vi "Menu.vi"() -> ()   [LabVIEW 2025]
panel:
  in  "Tab Control":enum32{"Page 1", "Page 2"}(tab)
  in  "Start Game":bool
  in  "Exit":bool
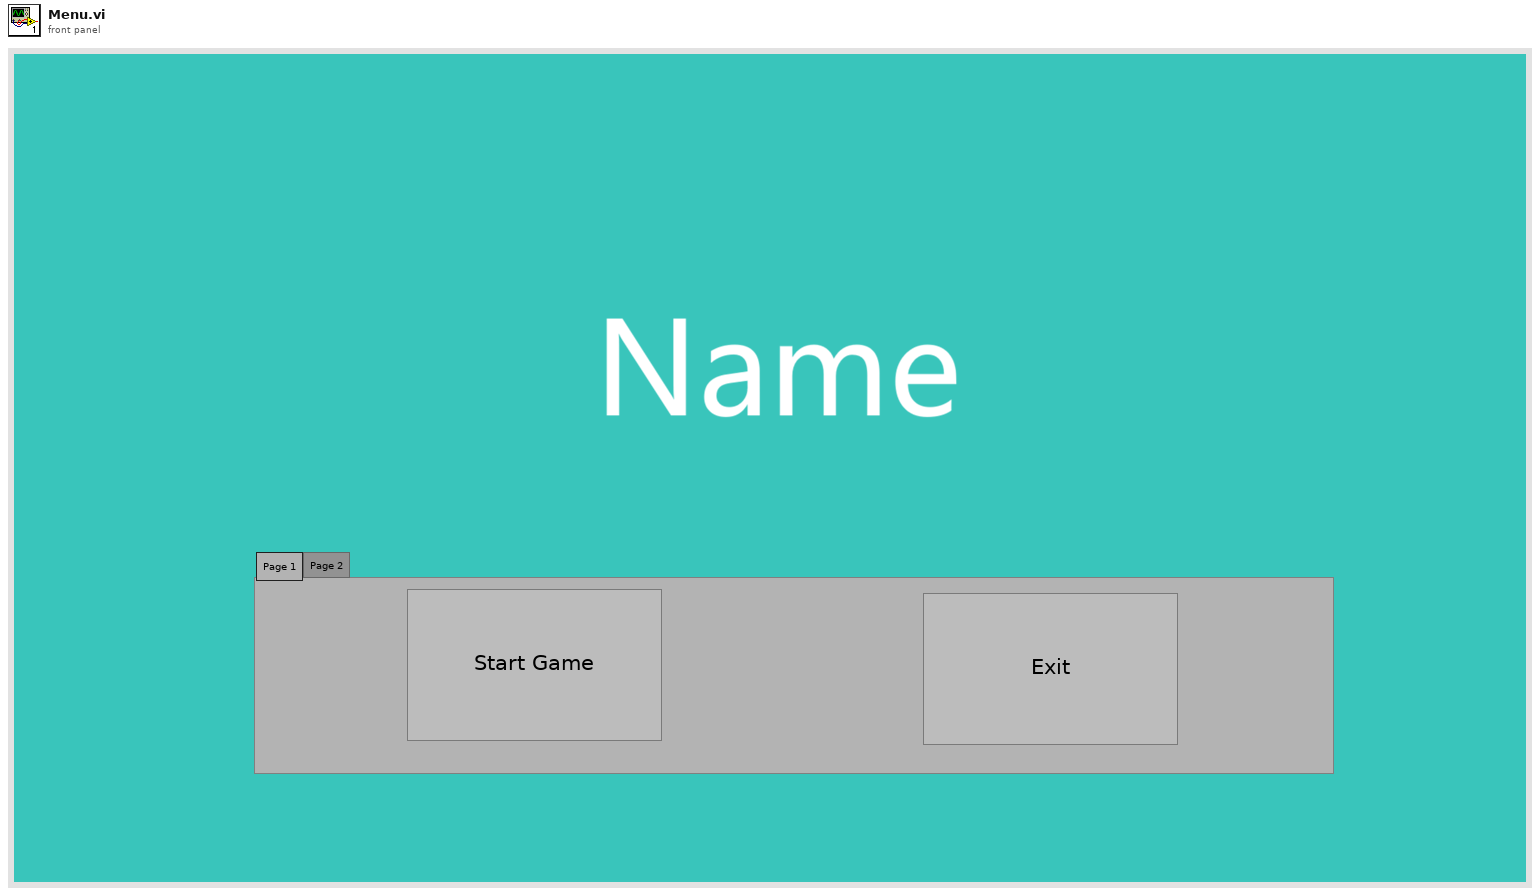
[diagram p1: front panel]
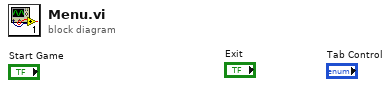
[diagram p0: block diagram]
diagram:
